vi "TESTE.vi"() -> ()   [LabVIEW 2018]
uses:
  CCDCamera/CCDCamera.lvclass
  <userlib>/atmcd32d.llb/Shutter_mode typedef.ctl
  <userlib>/atmcd32d.llb/ReadMode_mode typedef.ctl
  <userlib>/atmcd32d.llb/AcquisitionMode_mode typedef.ctl
  <userlib>/atmcd32d.llb/FITS_type typedef.ctl
  Simulated_CCD_Camera/Simulated_CCD_Camera.lvclass
  Interface/Interface.lvclass
  <userlib>/gfitsio/gfitsio.lvlib
  <userlib>/gfitsio/cfitsio-bitpix.ctl
  <userlib>/gfitsio/gfitsio-write-image-subset-i32-1d.vi
  C:/Users/observer/Desktop/SPARC4_ACS/SPARC4_ACS/Simulated_CCD_Camera/Simulated_CCD_Camera.lvclass
panel:
  out "return value":i32
  out "error out":errorcluster
  in  "Previous SET parameters":T1
  in  "Previous CCD Config":T5={"PREAMP"=enum."Gain 1", "READOUT_RATE"=enum."1 MHz", "EM_GAIN"=2, "VBIN"=1, "INITIAL_LINE"=1, "INITIAL_COLUMN"=1, "FINAL_LINE"=1024, "FINAL_COLUMN"=1024, "TRIGGER_MODE"=enum."Internal", "HBIN"=1, "SHUTTER_TTL"=enum."TTL Low", "SHUTTER_MODE"=enum."Close", "SHUTTER_OPENING_TIME"=50, "SHUTTER_CLOSING_TIME"=50, "VERTICAL_SHIFT_SPEED"=3, "READ_MODE"=enum."Image", "FRAME_TRANSFER"=TRUE, "VERTICAL_CLOCK_VOLTAGE"=enum."0", "ACQUISITION_MODE"=enum."Kinetics", "AD_CHANNEL"=0, "EM_MODE"=enum."Electron Multiplying"}
  in  "CCDCamera.lvclass":refnum<class "CCDCamera.lvclass">
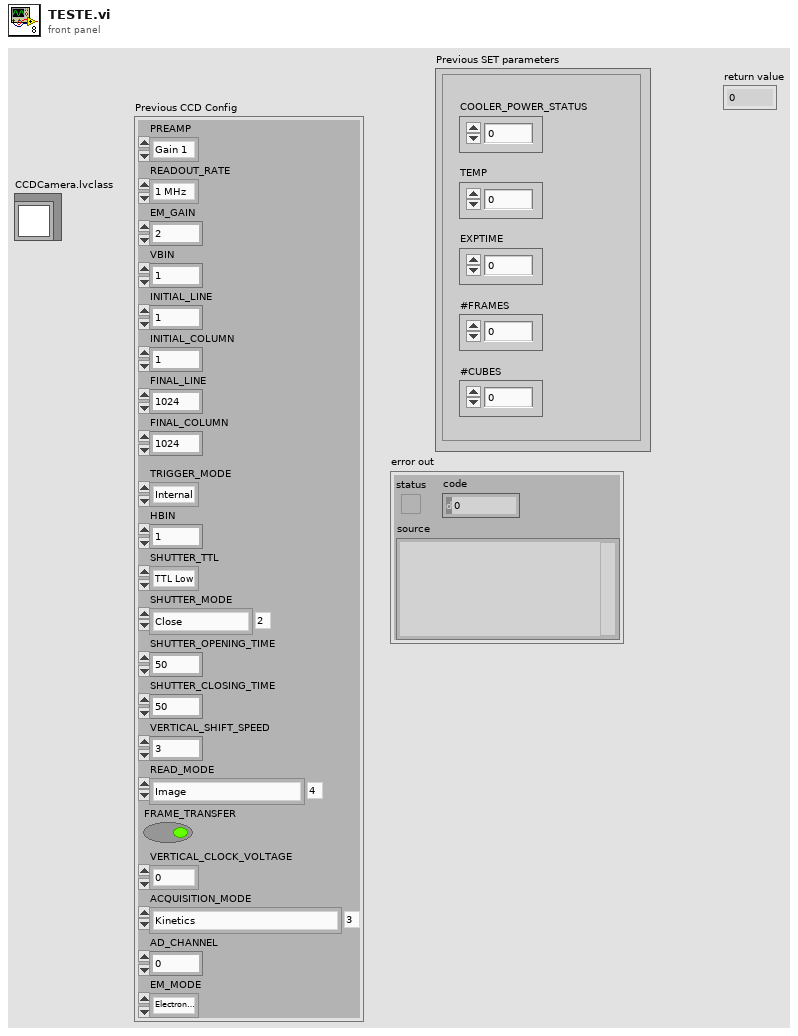
[diagram p1: front panel]
types:
  T1 = cluster{"COOLER_POWER_STATUS":u16, "TEMP":i32, "EXPTIME":dbl, "#FRAMES":u32, "#CUBES":u32}
  T2 = typedef "Shutter_mode typedef.ctl" = enum16{"Auto", "Open", "Close", "N/A (3)", "Open FVB Series", "Open Any Series"}
  T3 = typedef "ReadMode_mode typedef.ctl" = enum16{"Full Vertical Binning", "Multi-Track", "Random-Track", "Single-Track", "Image"}
  T4 = typedef "AcquisitionMode_mode typedef.ctl" = enum16{"Reserved (0)", "Single Scan", "Accumulate", "Kinetics", "Fast Kinetics", "Run Till Abort", "Reserved (6)", "Reserved (7)", "Reserved (8)", "Time Delayed Integration"}
  T5 = cluster{"PREAMP":enum16{"Gain 1", "Gain 2"}, "READOUT_RATE":enum16{"30 MHz", "20 MHz", "10 MHz", "1 MHz"}, "EM_GAIN":u16, "VBIN":u16, "INITIAL_LINE":u16, "INITIAL_COLUMN":u16, "FINAL_LINE":u16, "FINAL_COLUMN":u16, "TRIGGER_MODE":enum16{"Internal", "External", "N/A", "N/A_1", "N/A_2", "N/A_3", "External Start"}, "HBIN":u16, "SHUTTER_TTL":enum16{"TTL Low", "TTL High"}, "SHUTTER_MODE":T2, "SHUTTER_OPENING_TIME":u16, "SHUTTER_CLOSING_TIME":u16, "VERTICAL_SHIFT_SPEED":u16, "READ_MODE":T3, "FRAME_TRANSFER":bool, "VERTICAL_CLOCK_VOLTAGE":enum16{"0", "+1", "+2", "+3", "+4"}, "ACQUISITION_MODE":T4, "AD_CHANNEL":u16, "EM_MODE":enum16{"Electron Multiplying", "Conventional"}}
  T6 = typedef "FITS_type typedef.ctl" = enum16{"Unsigned 16", "Unsigned 32", "Signed 16", "Signed 32", "Float"}
  T7 = enum16{"open", "open or create", "create", "create or replace"}
  T8 = enum16{"open", "open or create", "create or replace", "create", "open (read only)"}
  T9 = typedef "gfitsio.lvlib/cfitsio-bitpix.ctl" = i32
  T10 = typedef "gfitsio.lvlib/gfitsio-refnum.ctl" = refnum<k1>
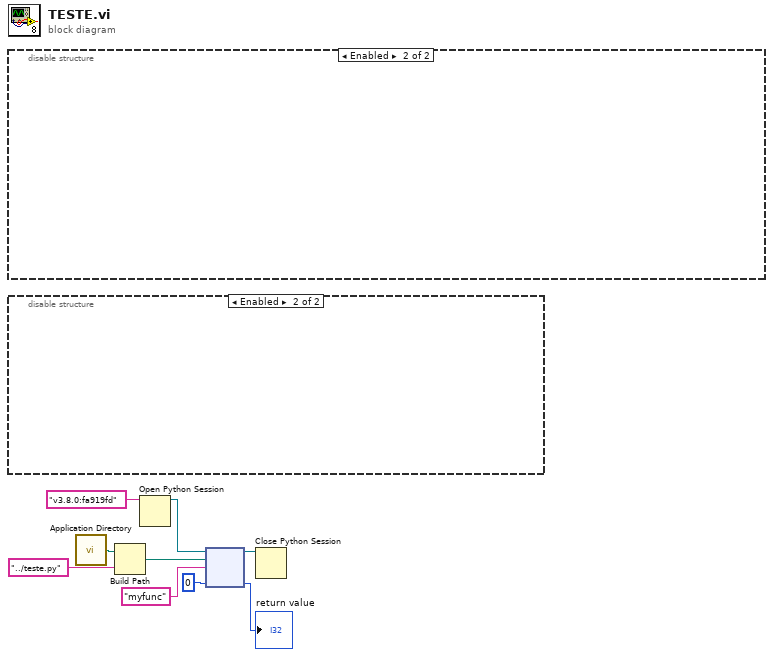
[diagram p0: block diagram]
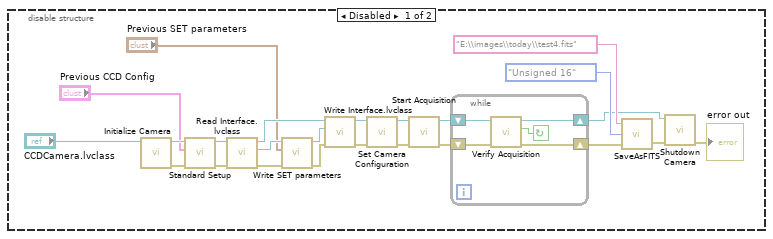
[diagram p2: hidden frame]
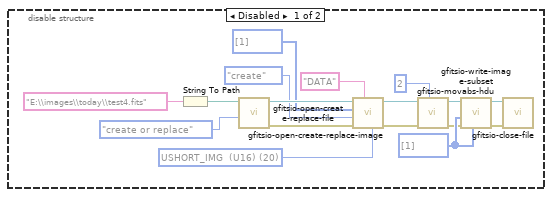
[diagram p3: hidden frame]
diagram:
  n1 = disable-structure shown="Enabled" {
    frame Disabled {
      n2 = call-dynamic "Initialize Camera.vi"("CCDCamera in"="CCDCamera.lvclass") -> ("error out"=w30:errorcluster, "CCDCamera out"=w33:refnum<class "CCDCamera.lvclass">)  [unwired: 9 in]
      n3 = call-dynamic "Standard Setup.vi"("error in (no error)"=w30, "Previous CCD Config"="Previous CCD Config", "CCDCamera in"=w33) -> ("error out"=w21:errorcluster, "CCDCamera out"=w25:refnum<class "CCDCamera.lvclass">)  [unwired: 7 in]
      n4 = call "Read Interface.lvclass.vi"("error in (no error)"=w21, "Simulated_CCD_Camera in"=w25) -> ("error out"=w20:errorcluster, "Interface.lvclass"=w17:refnum<class "Interface.lvclass">, "Simulated_CCD_Camera out"=w24:refnum<class "CCDCamera.lvclass">)  [unwired: 7 in]
      n5 = call "Write SET parameters.vi"("error in (no error)"=w20, "SET parameters"="Previous SET parameters", "Interface in"=w17) -> ("error out"=w19:errorcluster, "Interface out"=w18:refnum<class "Interface.lvclass">)  [unwired: 7 in]
      n6 = call "Write Interface.lvclass.vi"("error in (no error)"=w19, "Interface.lvclass"=w18, "Simulated_CCD_Camera in"=w24) -> ("error out"=w22:errorcluster, "Simulated_CCD_Camera out"=w23:refnum<class "CCDCamera.lvclass">)  [unwired: 7 in]
      n7 = call-dynamic "Set Camera Configuration.vi"("error in (no error)"=w22, "CCDCamera in"=w23) -> ("error out"=w26:errorcluster, "CCDCamera out"=w27:refnum<class "CCDCamera.lvclass">)  [unwired: 8 in]
      n8 = call-dynamic "Start Acquisition.vi"("error in (no error)"=w26, "CCDCamera in"=w27) -> ("error out"=w31:errorcluster, "CCDCamera out"=w32:refnum<class "CCDCamera.lvclass">)  [unwired: 8 in]
      n9 = while {
        shift-right: [w37] -> w11
        shift-left: w32 -> [w38]
        shift-right: [w34] -> w10
        shift-left: w31 -> [w36]
        stop <- w35 continue-if-true
        n10 = call-dynamic "Verify Acquisition.vi"("error in (no error)"=w36, "CCDCamera in"=w38) -> ("error out"=w34:errorcluster, "Acquiring"=w35:bool, "CCDCamera out"=w37:refnum<class "CCDCamera.lvclass">)  [unwired: 7 in]
      }
      n11 = call <userlib>:"SaveAsFITS.vi"("error in (no error)"=w10, "FITS_type"=FITS_type_typedef."Unsigned 16", "path"="E:\\images\\today\\test4.fits") -> ("error out"=w12:errorcluster)  [unwired: 1 out]
      n12 = call-dynamic "Shutdown Camera.vi"("error in (no error)"=w12, "CCDCamera in"=w11) -> ("error out"=→"error out":errorcluster)  [unwired: 8 in, 1 out]
    }
    frame Enabled {
    }
  }
  n13 = disable-structure shown="Enabled" {
    frame Disabled {
      w47 = T9 20 items=["<invalid type>"=0, "BYTE_IMG  (U8)"=8, "SHORT_IMG  (I16)"=16, "USHORT_IMG  (U16)"=20, "LONG_IMG  (I32)"=32, "ULONG_IMG  (U32)"=40, "FLOAT_IMG  (SGL)"=-32, "DOUBLE_IMG  (DBL)"=-64] ("image data type")
      w50 = i32[] [1] ("fpixel")
      n14 = String To Path(string="E:\\images\\today\\test4.fits" ("path")) -> (path=w54:path)
      n15 = call <userlib>:"gfitsio-open-create-replace-file.vi"("function (open)"=T8."create or replace", "file path (dialog if empty)"=w54) -> ("error out"=w49:errorcluster, "gfits refnum"=w48:T10)  [unwired: 7 in, 1 out]
      n16 = call <userlib>:"gfitsio-open-create-replace-image.vi"("image data type"=w47, "hdu name (dialog if empty)"="DATA", "error in (no error)"=w49, "function (create or replace)"=T7."create", "naxes"=i32[] [1], "gfits refnum"=w48) -> ("error out"=w43:errorcluster, "dup gfits refnum"=w40:T10)  [unwired: 3 in, 1 out]
      n17 = call <userlib>:"gfitsio-movabs-hdu.vi"("hdunum"=2, "error in (no error)"=w43, "gfits refnum"=w40) -> ("error out"=w42:errorcluster, "dup gfits refnum"=w41:T10)  [unwired: 6 in, 1 out]
      n18 = call-poly <userlib>:"gfitsio-write-image-subset.vi"("fpixel"=w50, "error in (no error)"=w42, "data"=w50, "gfits refnum"=w41) -> ("error out"=w51:errorcluster, "dup gfits refnum"=w52:T10)  [unwired: 6 in]
      n19 = call <userlib>:"gfitsio-close-file.vi"("error in (no error)"=w51, "gfits refnum"=w52) -> ()  [unwired: 8 in, 2 out]
    }
    frame Enabled {
    }
  }
  n20 = call <vilib>:"Application Directory.vi"() -> ("Application Directory"=w9:path)
  n21 = Build Path(base path=w9, name or relative path="../teste.py") -> (appended path=w7:path)
  n22 = Open Python Session(python version="v3.8.0:fa919fd" ("Python version")) -> (session out=w2:refnum<k35>)  [unwired: 2 in, 1 out]
  n23 = node(w2, w7, "myfunc" ("function name"), 0) -> (w3:refnum<k35>, →"return value":i32)  [unwired: 1 in, 3 out]
  n24 = Close Python Session(session in=w3) -> ()  [unwired: 1 in, 1 out]
